vi "Bluetooth inicjalizacja.vi"(11 "time limit ms (10000)":i32) -> (0 "error out":errorcluster, 1 "service list":T1(array[cluster]), 2 "Number of devices":u16, 3 "Bluetooth Network Connection out":refnum<k31>, 4 "channel":u16, 5 "Device Name":string)   [LabVIEW 2013]
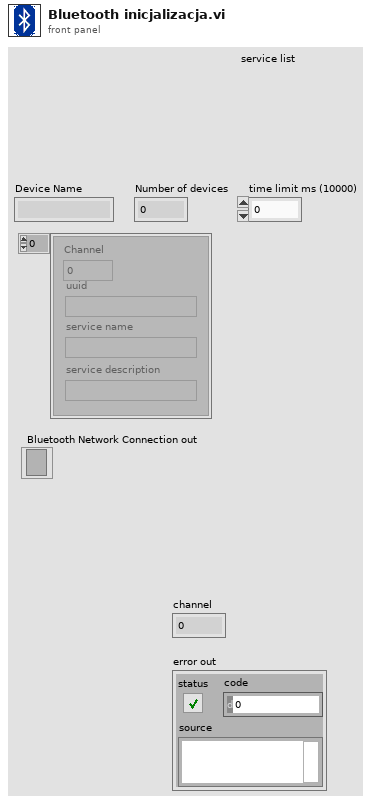
[diagram p1: front panel]
types:
  T1 = cluster{"Channel":u16, "uuid":string, "service name":string, "service description":string}[]
  T2 = cluster{"Address":string, "Device Name":string}[]
  T3 = cluster{"channel":u16, "uuid":string, "service name":string, "service description":string}[]
  T4 = cluster{"channel":u16, "uuid":string, "service name":string, "service description":string}
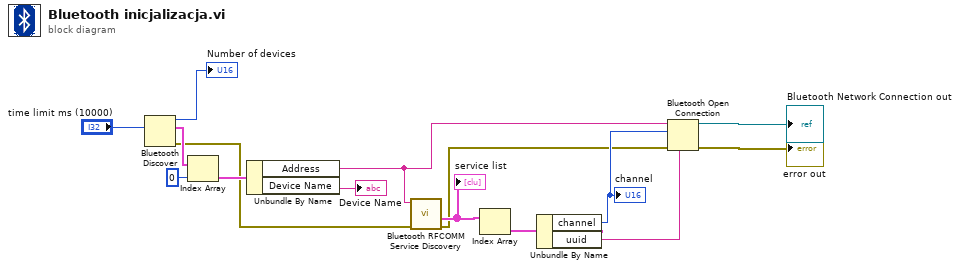
[diagram p0: block diagram]
diagram:
  n1 = Bluetooth Discover(10:"time limit ms (10000)") -> (0:w2:errorcluster, 2:w5:T2, 3:→"Number of devices":u16)  [unwired: 1 in]
  n2 = Index Array(array=w5, index=0) -> (element=w7:cluster{"Address":string, "Device Name":string})
  n3 = Unbundle By Name(w7) -> ("Address"=w13:string, "Device Name"=→"Device Name":string)
  n4 = call <vilib>:"Bluetooth RFCOMM Service Discovery.vi"("error in (no error)"=w2, "address in"=w13) -> ("error out"=w1:errorcluster, "service list"=w9:T3)  [unwired: 2 in, 2 out]
  "service list" <- w9
  n5 = Index Array(array=w9) -> (element=w10:T4)  [unwired: 1 in]
  n6 = Unbundle By Name(w10) -> ("channel"=w12:u16, "uuid"=w11:string)
  "channel" <- w12
  n7 = Bluetooth Open Connection(6:w11, 8:w1, 10:w12, 11:w13) -> (0:→"error out":errorcluster, 3:→"Bluetooth Network Connection out":refnum<k31>)  [unwired: 1 in]
